vi "Coffee Machine.vi"(11 "Error In":errorcluster) -> (15 "Error Out":errorcluster)   [LabVIEW 2020]
uses:
  Typedef/Queue_Operations.ctl
  Typedef/Coffee Machine Data.ctl
  <vilib>/Utility/config.llb/Read Key (Boolean).vi
  <vilib>/Utility/config.llb/Read Key (I32).vi
  <vilib>/Utility/config.llb/NI_LVConfig.lvlib
panel:
  in  "Power On":bool
  in  "Type":i32(knob) scale=0.0..2.0
  out "Total Cups":i32
  out "Elapsed Time":i32
  out "Dispensing":bool
  out "Brewing":bool
  out "Grinding":bool
  out "Heating":bool
  out "Purging":bool
  out "Low Milk":bool
  out "Low Bean":bool
  out "Low Water":bool
  in  "Dispenser":dbl(slide) scale=0.0..60.0
  in  "Chamber":dbl(slide) scale=0.0..60.0
  out "Milk Level":i32(slide)=60 scale=0.0..100.0
  out "Bean Level":i32(slide)=60 scale=0.0..100.0
  out "Water Level":i32(slide)=60 scale=0.0..100.0
  in  "1 Carafe":bool
  in  "1 Cup":bool
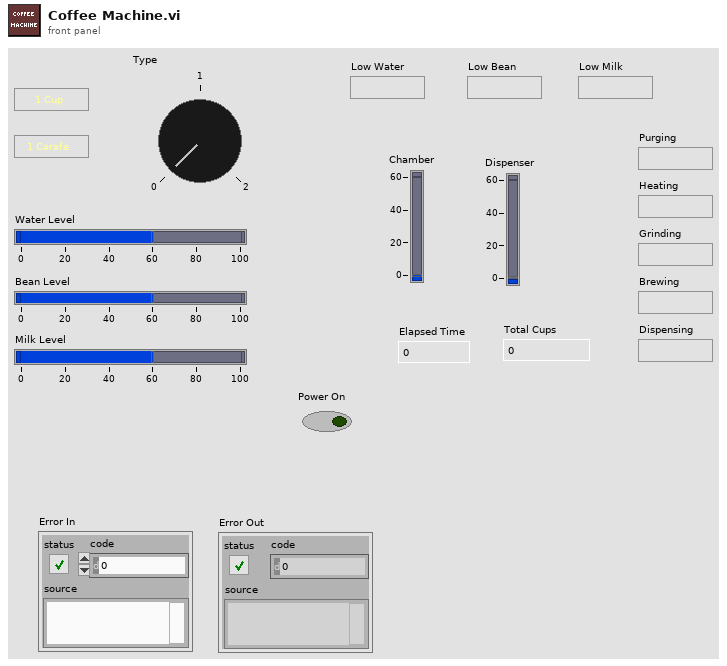
[diagram p1: front panel]
types:
  T1 = typedef "Coffee Machine Data.ctl" = cluster{"Proper Shutdown?":bool, "Purging":bool, "Heating":bool, "Grinding":bool, "Brewing":bool, "Dispensing":bool, "Total Cups":i32, "Elapsed Time":i32, "Start Time":dbl, "Power On":bool, "Start Timer":bool, "Low Water":bool, "Low Bean":bool, "Low Milk":bool, "Water Level":i32, "Bean Level":i32, "Milk Level":i32, "Type":i32, "Selected Units":i32}
  T2 = typedef "Queue_Operations.ctl" = enum16{"Create", "Enqueue", "Enqueue N", "Dequeue", "Enstack", "Flush", "Release"}
  T3 = typedef "NI_LVConfig.lvlib/Config Data RefNum.ctl" = refnum<k1>
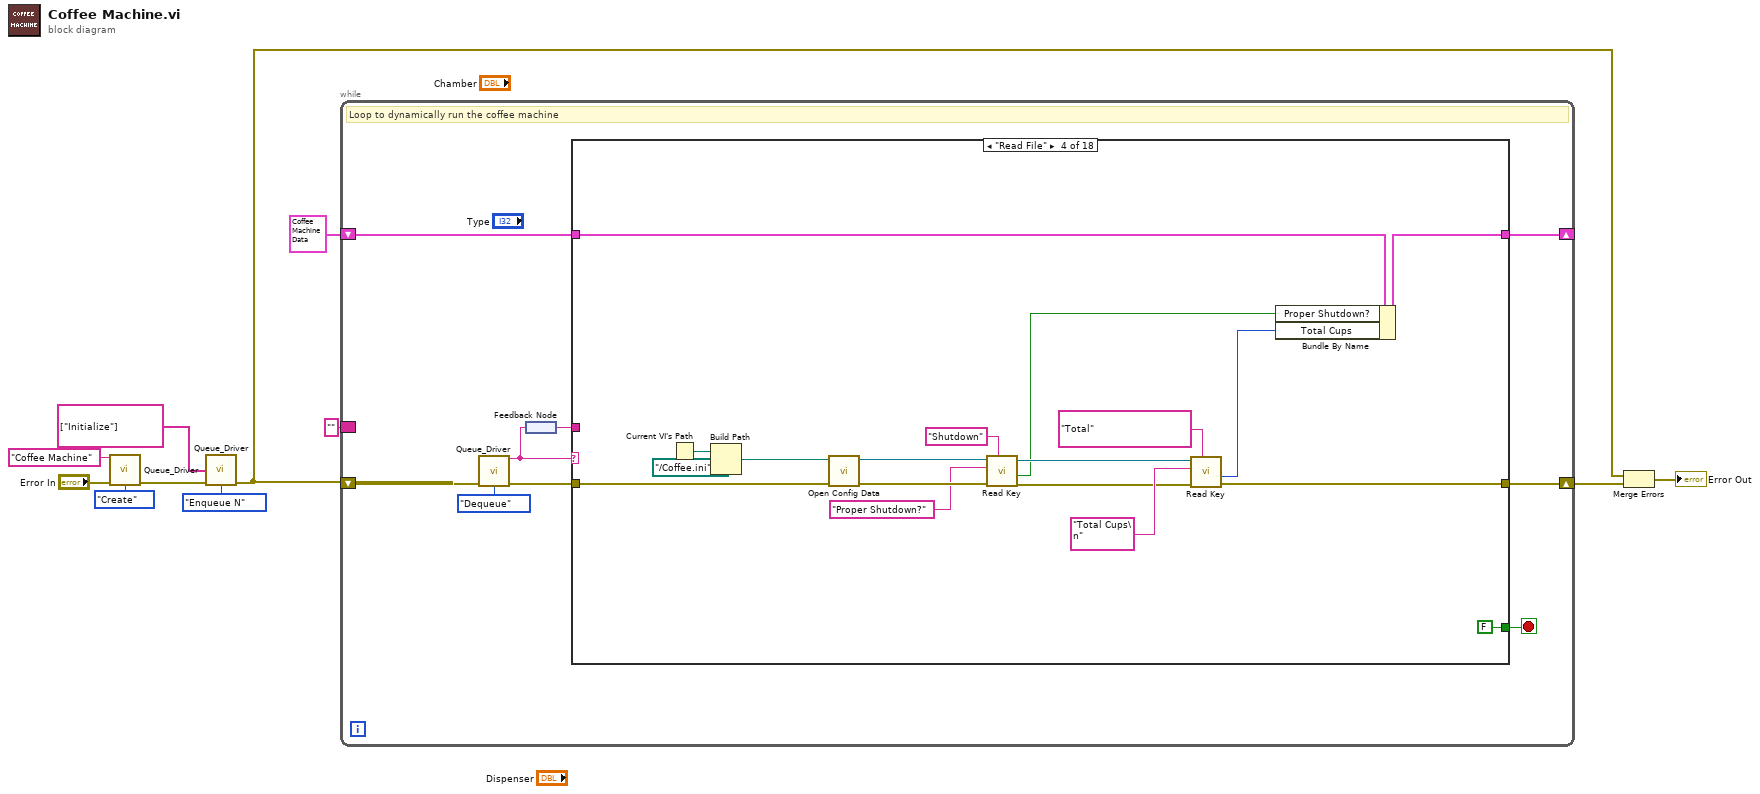
[diagram p0: block diagram]
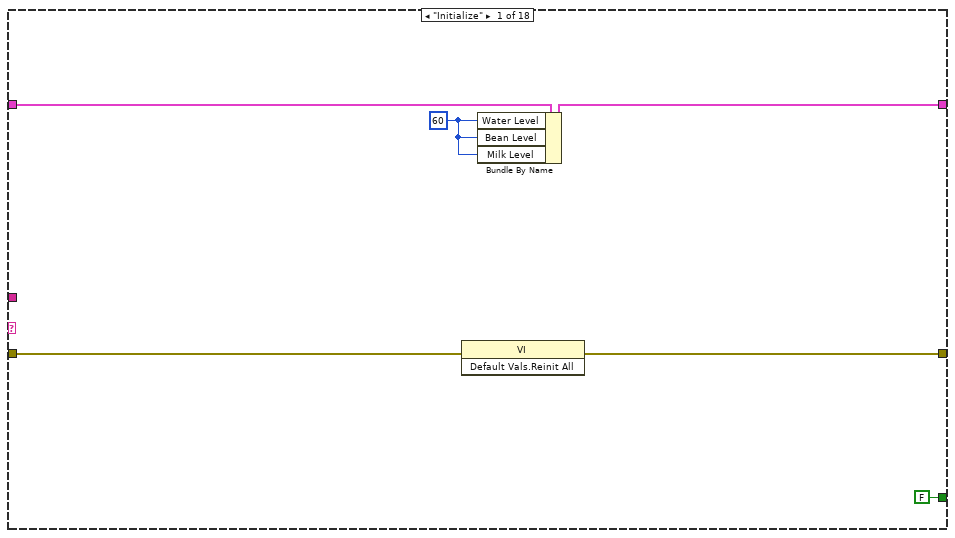
[diagram p2: hidden frame]
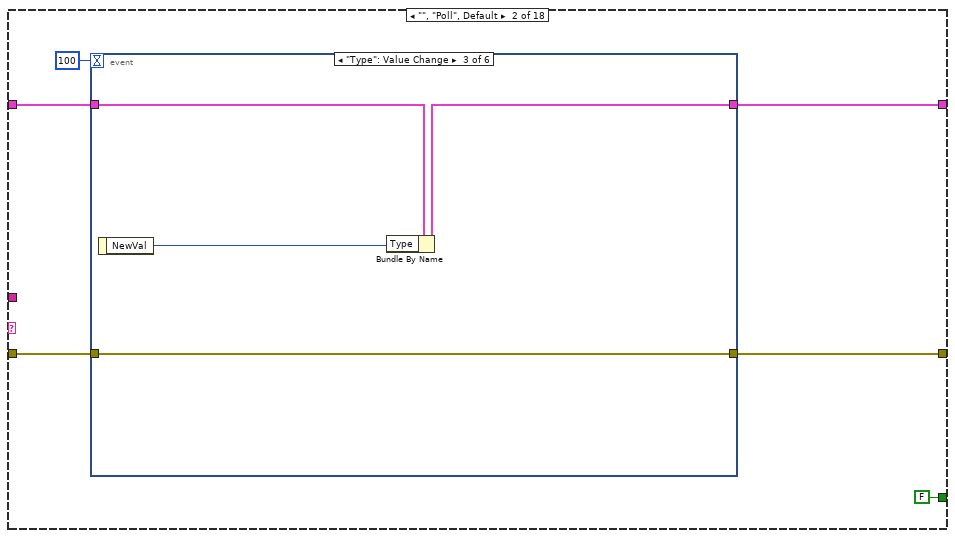
[diagram p3: hidden frame]
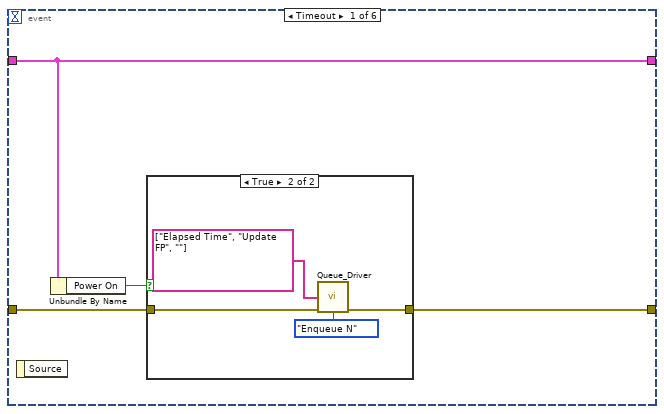
[diagram p4: hidden frame]
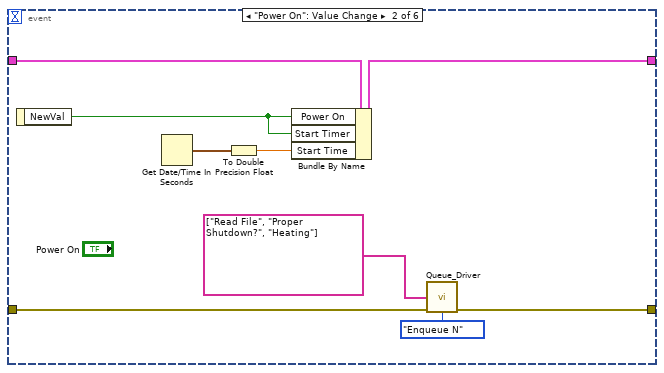
[diagram p6: hidden frame]
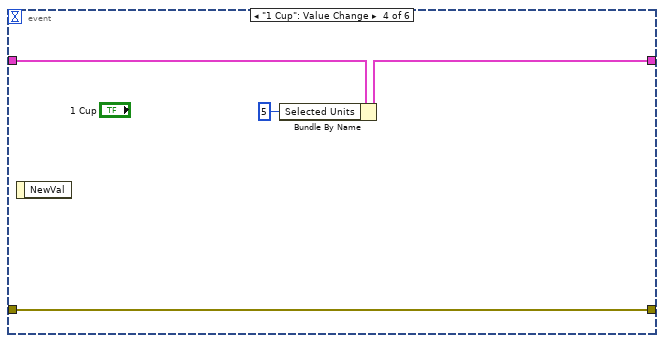
[diagram p7: hidden frame]
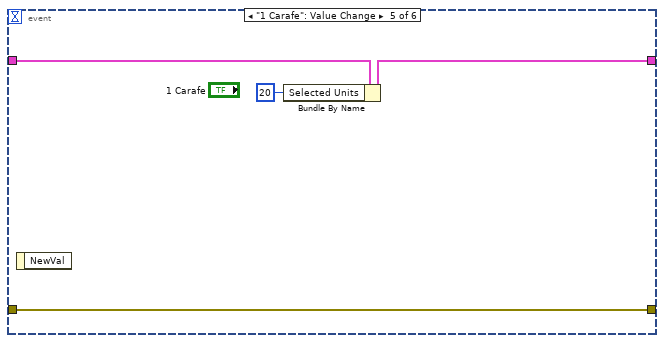
[diagram p8: hidden frame]
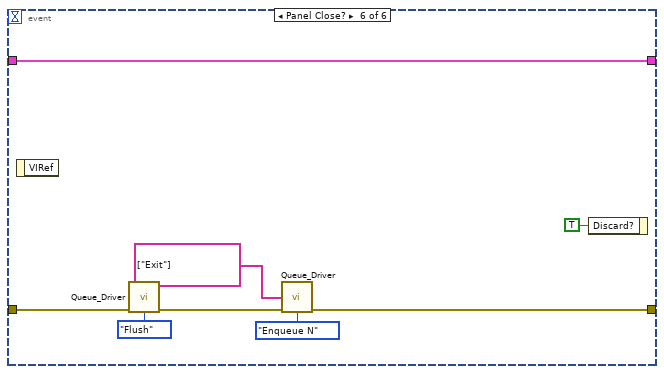
[diagram p9: hidden frame]
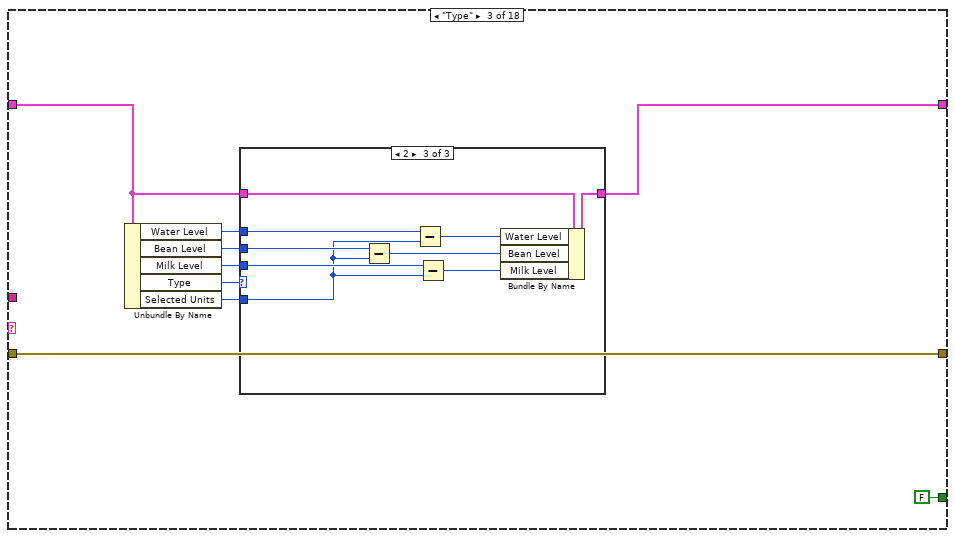
[diagram p10: hidden frame]
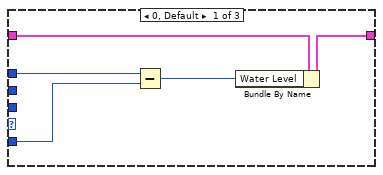
[diagram p11: hidden frame]
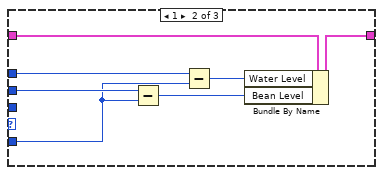
[diagram p12: hidden frame]
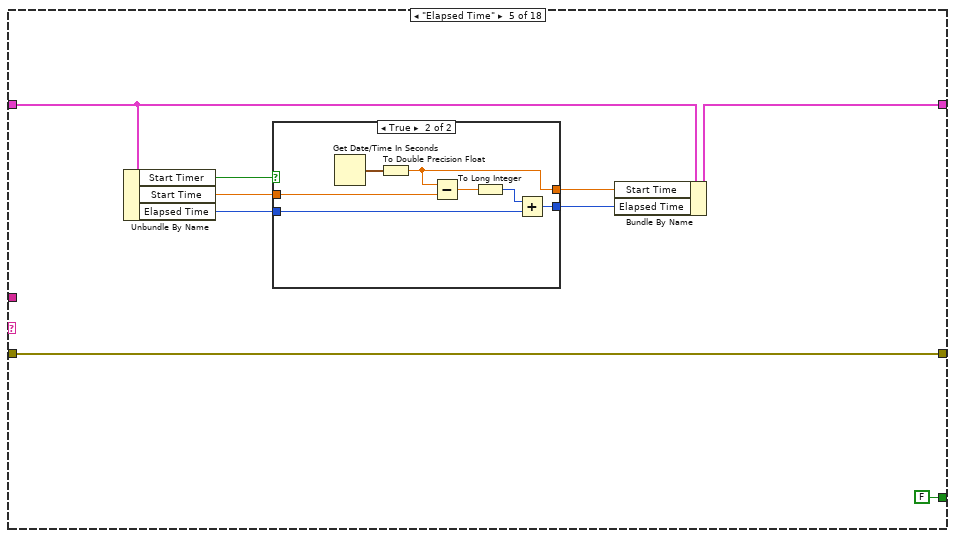
[diagram p13: hidden frame]
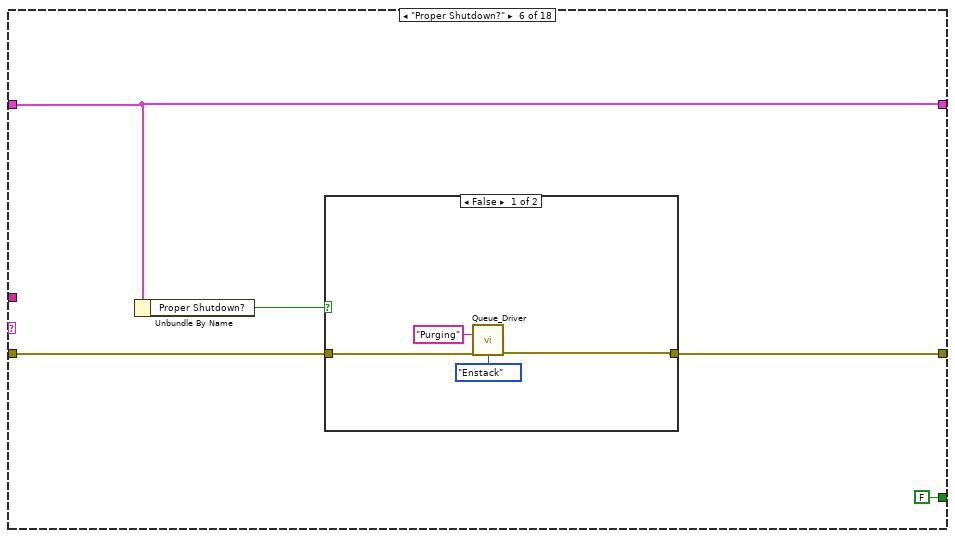
[diagram p15: hidden frame]
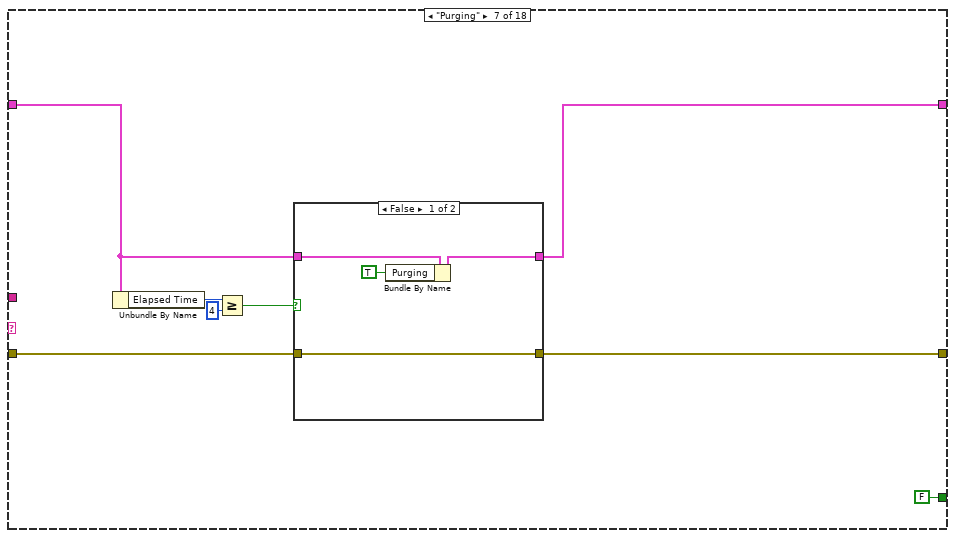
[diagram p17: hidden frame]
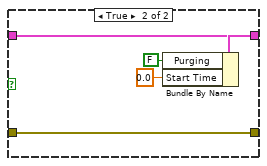
[diagram p18: hidden frame]
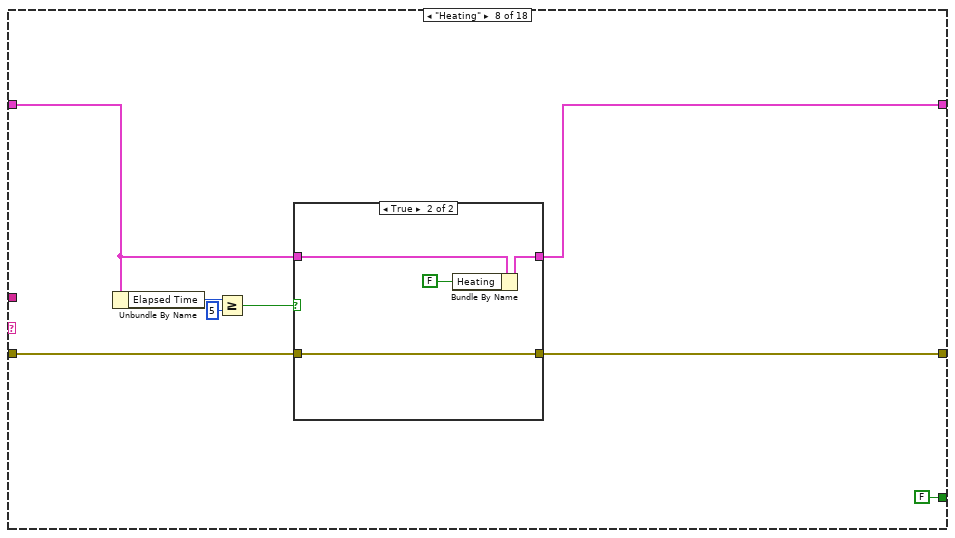
[diagram p19: hidden frame]
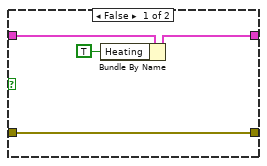
[diagram p20: hidden frame]
diagram:
  n1 = call "Queue_Driver.vi"("Queue Name"="Coffee Machine", "Error In"="Error In", "Queue Operation"=Queue_Operations."Create") -> ("Error Out"=w6:errorcluster)  [unwired: 11 in, 1 out]
  n2 = call "Queue_Driver.vi"("Array of States"=string[] ["Initialize"], "Error In"=w6, "Queue Operation"=Queue_Operations."Enqueue N") -> ("Error Out"=w4:errorcluster)  [unwired: 11 in, 1 out]
  n3 = while {
    shift-right: [w20] -> w11
    shift-left: w4 -> [w18]
    border: "" ("Dequeue Element") -> [_]
    shift-right: [w12] -> _
    shift-left: T1 {"Proper Shutdown?"=FALSE, "Purging"=FALSE, "Heating"=FALSE, "Grinding"=FALSE, "Brewing"=FALSE, "Dispensing"=FALSE, "Total Cups"=0, "Elapsed Time"=0, "Start Time"=0.0, "Power On"=FALSE, "Start Timer"=FALSE, "Low Water"=FALSE, "Low Bean"=FALSE, "Low Milk"=FALSE, "Water Level"=60, "Bean Level"=60, "Milk Level"=60, "Type"=0, "Selected Units"=0} -> [w13]
    stop <- w14 stop-if-true
    # "Loop to dynamically run the coffee machine"
    n4 = call "Queue_Driver.vi"("Error In"=w18, "Queue Operation"=Queue_Operations."Dequeue") -> ("Dequeue Element"=w15:string, "Error Out"=w17:errorcluster)  [unwired: 12 in]
    n5 = feedback-in #1(w15) -> ()
    n6 = feedback #1() -> (w16:string)
    n7 = case shown="\"Read File\"" w15 {
      tunnel: w17 -> [w26 w32 w79 w118 w127 w140 w152 w169 w185 w196 w202 w213 w222 w231 w253 w256 w269 w280]
      tunnel: [w25 w31 w79 w106 w127 w139 w151 w168 w184 w196 w201 w212 w221 w230 w253 w256 w262 w279] -> w20
      tunnel: w16 -> [_ _ _ _ _ _ _ _ _ _ _ _ _ _ _ _ w261 _]
      tunnel: [FALSE FALSE FALSE FALSE FALSE FALSE FALSE FALSE FALSE FALSE FALSE FALSE FALSE FALSE FALSE FALSE FALSE TRUE] -> w14
      tunnel: w13 -> [w23 w28 w73 w104 w126 w137 w147 w164 w180 w195 w197 w217 w226 w235 w252 w255 w257 w277]
      tunnel: [w22 w27 w72 w103 w123 w137 w148 w165 w181 w195 w198 w217 w226 w235 w252 w255 w257 w277] -> w12
      frame "Initialize" {
        w21 = 60 ("Water Level")
        n8 = invoke class="VI" method="Default Vals.Reinit All"(error in=w26) -> (error out=w25:errorcluster)  [unwired: 2 in, 2 out]
        n9 = Bundle By Name(cluster=w23, "Water Level"=w21, "Bean Level"=w21, "Milk Level"=w21) -> (w22:T1)
      }
      frame "", "Poll", Default {
        n10 = event shown="[2] \"Type\": Value Change" {
          selector: _ -> [_ _ _ _ _ _]
          dyn-events: _ -> [_ _ _ _ _ _]
          timeout: 100 -> [_ _ _ _ _ _]
          tunnel: w32 -> [w36 w49 w54 w58 w62 w67]
          tunnel: [w35 w48 w54 w58 w62 w64] -> w31
          tunnel: w28 -> [w34 w47 w53 w57 w61 w70]
          tunnel: [w34 w45 w52 w56 w60 w70] -> w27
          event Timeout {
            n11 = event-data() -> ()  [unwired: 1 in, 1 out]
            n12 = Unbundle By Name(w34) -> ("Power On"=w33:bool)
            n13 = case shown="True" w33 {
              tunnel: w36 -> [w37 w41]
              tunnel: [w37 w40] -> w35
              frame False {
              }
              frame True {
                n14 = call "Queue_Driver.vi"("Array of States"=string[] ["Elapsed Time", "Update FP", ""], "Error In"=w41, "Queue Operation"=Queue_Operations."Enqueue N") -> ("Error Out"=w40:errorcluster)  [unwired: 11 in, 1 out]
              }
            }
          }
          event "Power On": Value Change {
            n15 = event-data() -> ("NewVal"=w44:bool)  [unwired: 1 in]
            n16 = Get Date/Time In Seconds() -> (seconds since 1Jan1904=w43:timestamp)
            n17 = To Double Precision Float(number=w43) -> (double precision float=w42:dbl)
            n18 = Bundle By Name(cluster=w47, "Power On"=w44, "Start Timer"=w44, "Start Time"=w42) -> (w45:T1)
            n19 = call "Queue_Driver.vi"("Array of States"=string[] ["Read File", "Proper Shutdown?", "Heating"], "Error In"=w49, "Queue Operation"=Queue_Operations."Enqueue N") -> ("Error Out"=w48:errorcluster)  [unwired: 11 in, 1 out]
          }
          event "Type": Value Change {
            n20 = event-data() -> ("NewVal"=w51:i32)  [unwired: 1 in]
            n21 = Bundle By Name(cluster=w53, "Type"=w51) -> (w52:T1)
          }
          event "1 Cup": Value Change {
            n22 = event-data() -> ()  [unwired: 1 in, 1 out]
            n23 = Bundle By Name(cluster=w57, "Selected Units"=5) -> (w56:T1)
          }
          event "1 Carafe": Value Change {
            n24 = event-data() -> ()  [unwired: 1 in, 1 out]
            n25 = Bundle By Name(cluster=w61, "Selected Units"=20) -> (w60:T1)
          }
          event Panel Close? {
            n26 = event-data() -> ()  [unwired: 1 in, 1 out]
            n27 = call "Queue_Driver.vi"("Error In"=w67, "Queue Operation"=Queue_Operations."Flush") -> ("Error Out"=w65:errorcluster)  [unwired: 12 in, 1 out]
            n28 = call "Queue_Driver.vi"("Array of States"=string[] ["Exit"], "Error In"=w65, "Queue Operation"=Queue_Operations."Enqueue N") -> ("Error Out"=w64:errorcluster)  [unwired: 11 in, 1 out]
            n29 = event-data("Discard?"=TRUE) -> ()  [unwired: 1 in, 1 out]
          }
        }
      }
      frame "Type" {
        n30 = Unbundle By Name(w73) -> ("Water Level"=w77:i32, "Bean Level"=w76:i32, "Milk Level"=w75:i32, "Type"=w78:i32, "Selected Units"=w74:i32)
        n31 = case shown="2" w78 {
          tunnel: w77 -> [w84 w90 w99]
          tunnel: w76 -> [_ w91 w100]
          tunnel: w75 -> [_ _ w98]
          tunnel: w74 -> [w83 w89 w97]
          tunnel: [w81 w87 w95] -> w72
          tunnel: w73 -> [w82 w88 w96]
          frame 0, Default {
            n32 = Subtract(x=w84, y=w83) -> (x-y=w80:i32)
            n33 = Bundle By Name(cluster=w82, "Water Level"=w80) -> (w81:T1)
          }
          frame 1 {
            n34 = Subtract(x=w91, y=w89) -> (x-y=w85:i32)
            n35 = Subtract(x=w90, y=w89) -> (x-y=w86:i32)
            n36 = Bundle By Name(cluster=w88, "Water Level"=w86, "Bean Level"=w85) -> (w87:T1)
          }
          frame 2 {
            n37 = Subtract(x=w100, y=w97) -> (x-y=w93:i32)
            n38 = Subtract(x=w99, y=w97) -> (x-y=w94:i32)
            n39 = Subtract(x=w98, y=w97) -> (x-y=w92:i32)
            n40 = Bundle By Name(cluster=w96, "Water Level"=w94, "Bean Level"=w93, "Milk Level"=w92) -> (w95:T1)
          }
        }
      }
      frame "Read File" {
        n41 = Current VI's Path() -> (path=w115:path)
        n42 = Build Path(base path=w115, name or relative path=path "../Coffee.ini") -> (appended path=w116:path)
        n43 = call <vilib>:"Open Config Data.vi"("error in (no error)"=w118, "configuration file path"=w116) -> ("error out"=w117:errorcluster, "refnum"=w113:T3)  [unwired: 7 in, 1 out]
        n44 = call-poly <vilib>:"Read Key.vi"("section"="Shutdown", "error in (no error)"=w117, "key"="Proper Shutdown?", "refnum"=w113) -> ("error out"=w107:errorcluster, "value"=w102:bool, "refnum out"=w105:T3)  [unwired: 4 in, 1 out]
        n45 = call-poly <vilib>:"Read Key.vi"("section"="Total", "error in (no error)"=w107, "key"="Total Cups\n", "refnum"=w105) -> ("error out"=w106:errorcluster, "value"=w101:i32)  [unwired: 4 in, 2 out]
        n46 = Bundle By Name(cluster=w104, "Proper Shutdown?"=w102, "Total Cups"=w101) -> (w103:T1)
      }
      frame "Elapsed Time" {
        n47 = Unbundle By Name(w126) -> ("Start Timer"=w119:bool, "Start Time"=w125:dbl, "Elapsed Time"=w124:i32)
        n48 = case shown="True" w119 {
          tunnel: w125 -> [w129 w134]
          tunnel: w124 -> [w128 w133]
          tunnel: [w129 w132] -> w122
          tunnel: [w128 w131] -> w121
          frame False {
          }
          frame True {
            n49 = Get Date/Time In Seconds() -> (seconds since 1Jan1904=w136:timestamp)
            n50 = To Double Precision Float(number=w136) -> (double precision float=w132:dbl)
            n51 = Subtract(x=w132, y=w134) -> (x-y=w135:dbl)
            n52 = To Long Integer(number=w135) -> (32bit integer=w130:i32)
            n53 = Add(x=w130, y=w133) -> (x+y=w131:i32)
          }
        }
        n54 = Bundle By Name(cluster=w126, "Start Time"=w122, "Elapsed Time"=w121) -> (w123:T1)
      }
      frame "Proper Shutdown?" {
        n55 = Unbundle By Name(w137) -> ("Proper Shutdown?"=w141:bool)
        n56 = case shown="False" w141 {
          tunnel: [w143 w146] -> w139
          tunnel: w140 -> [w144 w146]
          frame False {
            n57 = call "Queue_Driver.vi"("State"="Purging", "Error In"=w144, "Queue Operation"=Queue_Operations."Enstack") -> ("Error Out"=w143:errorcluster)  [unwired: 11 in, 1 out]
          }
          frame True {
          }
        }
      }
      frame "Purging" {
        n58 = Unbundle By Name(w147) -> ("Elapsed Time"=w154:i32)
        n59 = Greater Or Equal?(x=w154, y=4) -> (x >= y?=w149:bool)
        n60 = case shown="False" w149 {
          tunnel: w152 -> [w158 w163]
          tunnel: [w158 w163] -> w151
          tunnel: [w156 w162] -> w148
          tunnel: w147 -> [w157 w161]
          frame False {
            n61 = Bundle By Name(cluster=w157, "Purging"=TRUE) -> (w156:T1)
          }
          frame True {
            n62 = Bundle By Name(cluster=w161, "Purging"=FALSE, "Start Time"=0.0) -> (w162:T1)
          }
        }
      }
      frame "Heating" {
        n63 = Unbundle By Name(w164) -> ("Elapsed Time"=w171:i32)
        n64 = Greater Or Equal?(x=w171, y=5) -> (x >= y?=w166:bool)
        n65 = case shown="True" w166 {
          tunnel: w169 -> [w174 w179]
          tunnel: [w174 w179] -> w168
          tunnel: [w173 w178] -> w165
          tunnel: w164 -> [w175 w177]
          frame False {
            n66 = Bundle By Name(cluster=w175, "Heating"=TRUE) -> (w173:T1)
          }
          frame True {
            n67 = Bundle By Name(cluster=w177, "Heating"=FALSE) -> (w178:T1)
          }
        }
      }
      frame "Brewing" {
        n68 = Unbundle By Name(w180) -> ("Elapsed Time"=w187:i32)
        n69 = Greater Or Equal?(x=w187, y=4) -> (x >= y?=w182:bool)
        n70 = case shown="True" w182 {
          tunnel: w185 -> [w188 w193]
          tunnel: [w188 w193] -> w184
          tunnel: [w189 w192] -> w181
          tunnel: w180 -> [w189 w191]
          frame False {
          }
          frame True {
            n71 = Bundle By Name(cluster=w191, "Brewing"=FALSE ("Heating")) -> (w192:T1)
          }
        }
      }
      frame "Grinding" {
      }
      frame "Dispensing" {
        n72 = Unbundle By Name(w197) -> ("Elapsed Time"=w204:i32)
        n73 = Greater Or Equal?(x=w204, y=5) -> (x >= y?=w199:bool)
        n74 = case shown="True" w199 {
          tunnel: w202 -> [w205 w210]
          tunnel: [w205 w210] -> w201
          tunnel: [w206 w209] -> w198
          tunnel: w197 -> [w206 w208]
          frame False {
          }
          frame True {
            n75 = Bundle By Name(cluster=w208, "Dispensing"=FALSE ("Heating")) -> (w209:T1)
          }
        }
      }
      frame "Milk Level" {
        n76 = Unbundle By Name(w217) -> ("Milk Level"=w216:i32)
        n77 = Less?(x=w216, y=30) -> (x < y?=w211:bool)
        n78 = case shown="False" w211 {
          tunnel: w213 -> [w218 w219]
          tunnel: [w218 w219] -> w212
          frame False {
          }
          frame True {
          }
        }
      }
      frame "Water Level" {
        n79 = Unbundle By Name(w226) -> ("Water Level"=w225:i32)
        n80 = Less?(x=w225, y=30) -> (x < y?=w220:bool)
        n81 = case shown="False" w220 {
          tunnel: w222 -> [w227 w228]
          tunnel: [w227 w228] -> w221
          frame False {
          }
          frame True {
          }
        }
      }
      frame "Bean Level" {
        n82 = Unbundle By Name(w235) -> ("Bean Level"=w234:i32)
        n83 = Less?(x=w234, y=30) -> (x < y?=w229:bool)
        n84 = case shown="False" w229 {
          tunnel: w231 -> [w236 w237]
          tunnel: [w236 w237] -> w230
          frame False {
          }
          frame True {
          }
        }
      }
      frame "Update FP" {
        n85 = Unbundle By Name(w252) -> ("Total Cups"=→"Total Cups":i32, "Elapsed Time"=→"Elapsed Time":i32, "Purging"=→"Purging":bool, "Heating"=→"Heating":bool, "Grinding"=→"Grinding":bool, "Brewing"=→"Brewing":bool, "Dispensing"=→"Dispensing":bool, "Low Water"=→"Low Water":bool, "Low Bean"=→"Low Bean":bool, "Low Milk"=→"Low Milk":bool, "Water Level"=→"Water Level":i32, "Bean Level"=→"Bean Level":i32, "Milk Level"=→"Milk Level":i32)
      }
      frame "Ingredient Check" {
      }
      frame "Error" {
        # "Displays the occurence of error and acts according to user input"
        n86 = Unbundle By Name(w269) -> ("code"=w268:i32, "source"=w267:string)
        n87 = Format Into String(format string="Error Occured in %s state\nError code is %d.\nThe source of the error is %s\nDo you want to continue? ", error in=w269, w261, w268, w267) -> (resulting string=w265:string, error out=w263:errorcluster)  [unwired: 1 in]
        n88 = Two Button Dialog(message=w265, 1:"Exit" ("F button name (\"Cancel\")"), 2:"Continue" ("T button name (\"OK\")")) -> (T button?=w264:bool)
        n89 = case shown="False" w264 {
          tunnel: w263 -> [w273 w276]
          tunnel: [w271 w276] -> w262
          frame False {
            # "Flushes the queue and enqueues the exit state to stop the VI running"
            n90 = call "Queue_Driver.vi"("Error In"=w273, "Queue Operation"=Queue_Operations."Flush") -> ("Error Out"=w272:errorcluster)  [unwired: 12 in, 1 out]
            n91 = call "Queue_Driver.vi"("Array of States"=string[] ["Exit"], "Error In"=w272, "Queue Operation"=Queue_Operations."Enqueue N") -> ("Error Out"=w271:errorcluster)  [unwired: 11 in, 1 out]
          }
          frame True {
            # "Continues the process"
          }
        }
      }
      frame "Exit" {
        n92 = call "Queue_Driver.vi"("Error In"=w280, "Queue Operation"=Queue_Operations."Release") -> ("Error Out"=w279:errorcluster)  [unwired: 12 in, 1 out]
      }
    }
  }
  n93 = Merge Errors(w4, w11) -> (→"Error Out":errorcluster)
